vi "Test Lookup API.vi"() -> (0 "test result":errorcluster)   [LabVIEW 2019, in "ANODE Tests.lvlib"]
uses:
  ANODE Tests.lvlib
  Base Class A.lvclass
  Class B-D.lvclass
  C:/Users/Nicholas Folse/Documents/workspace/github-tauterra.llc/ANODE/ANODE Tests/Lookup API/Class B.lvclass
  Class B.lvclass
  C:/Users/Nicholas Folse/Documents/workspace/github-tauterra.llc/ANODE/ANODE Tests/Lookup API/Base Class A.lvclass
  208e85c7-0cb6-4da8-adaf-c1f07bea2b81.vi
  350f7c64-ba5b-4f87-a26e-5058ffd36ae8.vi
  9f842d0e-53a4-4d11-badb-58d219860510.vi
  80fdccb2-9c7f-43c5-aac1-790debc25787.vi
  208e85c7-0cb6-4da8-adaf-c1f07bea2b81.vi/252e9e58-4af6-4f6d-a0ca-3bfdda4348ce.vi
  350f7c64-ba5b-4f87-a26e-5058ffd36ae8.vi/97c9d0db-94a5-468f-a424-c7048e2c2629.vi
  9f842d0e-53a4-4d11-badb-58d219860510.vi/c3dc75b2-7c32-4953-a8c5-a3642948c66d.vi
  ANODE/Lookup API/Services/Lookup Service/Lookup Service.lvclass
  Class C.lvclass
  1f8dec34-990c-434d-8cda-825a1ce43037.vi
panel:
  out "should have two instances of 'A'":bool
  out "error out":errorcluster
  out "pass?":bool
  out "object should be in set":bool
  out "B and B-C instance are both 'A's":bool
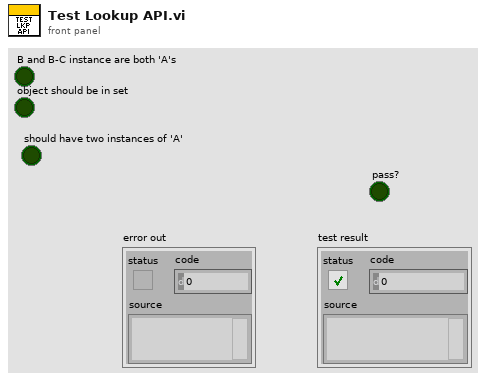
[diagram p1: front panel]
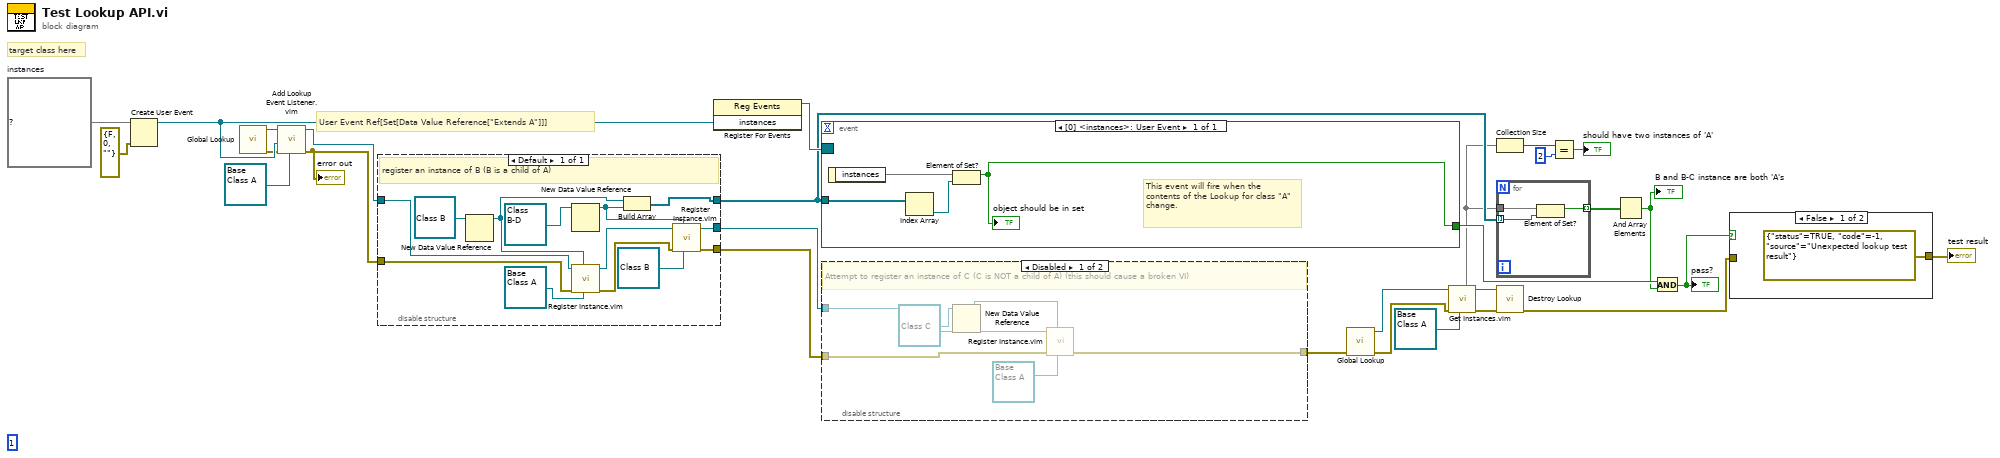
[diagram p0: block diagram]
diagram:
  (unwired) 1
  w13 = set{refnum<data-value>} {}  # instances
  # "User Event Ref[Set[Data Value Reference[\"Extends A\"]]]"
  # "target class here"
  n1 = Create User Event(user event datatype=w13, error in=errorcluster {"status"=FALSE, "code"=0, "source"=""} ("error in (no error)")) -> (user event=w12:refnum<user-event>)  [unwired: 1 out]
  n2 = call "Global Lookup.vi"() -> ("error out"=w8:errorcluster, "Global Lookup"=w15:refnum<data-value>)  [unwired: 10 in]
  n3 = call "Add Lookup Event Listener.vim"("Base Class (LabVIEW Object)"=refnum<class "Base Class A.lvclass"> refnum ("LVCOOOP Tests.lvlib:Base Class A.lvclass"), "error in (no error)"=w8, "user event"=w12, "Lookup Service in"=w15) -> ("error out"=w10:errorcluster, "Lookup Service out"=w11:refnum<data-value>)  [unwired: 6 in]
  "error out" <- w10
  n4 = disable-structure shown="Default" {
    disable-tunnel: w11 -> [w40]
    disable-tunnel: [w33] -> w27
    disable-tunnel: w10 -> [w39]
    disable-tunnel: [w32] -> w19
    disable-tunnel: [w29] -> w6
    frame Enabled {
      # "register an instance of B (B is a child of A)"
      n5 = New Data Value Reference(data value=refnum<class "Class B.lvclass"> refnum ("LVCOOOP Tests.lvlib:Class B.lvclass")) -> (data value reference=w31:refnum<data-value>)  [unwired: 1 in, 1 out]
      n6 = New Data Value Reference(data value=refnum<class "Class B-D.lvclass"> refnum ("LVCOOOP Tests.lvlib:Class B-D.lvclass")) -> (data value reference=w30:refnum<data-value>)  [unwired: 1 in, 1 out]
      n7 = call "Register Instance.vim"("Base Class (LabVIEW Object)"=refnum<class "Base Class A.lvclass"> refnum ("LVCOOOP Tests.lvlib:Base Class A.lvclass"), "Object Instance"=w31, "error in (no error)"=w39, "Lookup Service in"=w40) -> ("error out"=w36:errorcluster, "Lookup Service out"=w37:refnum<data-value>)  [unwired: 6 in]
      n8 = Build Array(w31, w30) -> (w29:refnum<data-value>[])
      n9 = call "Register Instance.vim"("Base Class (LabVIEW Object)"=refnum<class "Class B.lvclass"> refnum ("LVCOOOP Tests.lvlib:Class B.lvclass"), "Object Instance"=w30, "error in (no error)"=w36, "Lookup Service in"=w37) -> ("error out"=w32:errorcluster, "Lookup Service out"=w33:refnum<data-value>)  [unwired: 6 in]
    }
  }
  n10 = register-events(w12) -> (reference out=w28:refnum<event-registration>)  [unwired: 2 in, 1 out]
  n11 = event shown="[0] <instances>: User Event" {
    selector: w28 -> [_]
    dyn-events: _ -> [_]
    timeout: _ -> [_]
    tunnel: [w42] -> w24
    tunnel: w6 -> [w44]
    event User Event {
      # "This event will fire when the contents of the Lookup for class \"A\" change."
      n12 = event-data() -> ("instances"=w45:set{refnum<data-value>})  [unwired: 1 in]
      n13 = Index Array(array=w44) -> (element=w43:refnum<data-value>)  [unwired: 1 in]
      n14 = Element of Set?(10:w43, 11:w45) -> (3:w42:bool)
      "object should be in set" <- w42
    }
  }
  n15 = disable-structure shown="Disabled" {
    disable-tunnel: w27 -> [w51 _]
    disable-tunnel: w19 -> [w49 w52]
    disable-tunnel: [w46 w52] -> w18
    frame Disabled {
      # "Attempt to register an instance of C (C is NOT a child of A) (this should cause a broken VI)"
      n16 = New Data Value Reference(data value=refnum<class "Class C.lvclass"> refnum ("LVCOOOP Tests.lvlib:Class C.lvclass")) -> (data value reference=w47:refnum<data-value>)  [unwired: 1 in, 1 out]
      n17 = call "Register Instance.vim"("Base Class (LabVIEW Object)"=refnum<class "Base Class A.lvclass"> refnum ("LVCOOOP Tests.lvlib:Base Class A.lvclass"), "Object Instance"=w47, "error in (no error)"=w49, "Lookup Service in"=w51) -> ("error out"=w46:errorcluster)  [unwired: 6 in, 1 out]
    }
    frame Enabled {
    }
  }
  n18 = call "Global Lookup.vi"("error in (no error)"=w18) -> ("error out"=w17:errorcluster, "Global Lookup"=w16:refnum<data-value>)  [unwired: 9 in]
  n19 = call "Get Instances.vim"("Base Class (LabVIEW Object)"=refnum<class "Base Class A.lvclass"> refnum ("LVCOOOP Tests.lvlib:Base Class A.lvclass"), "error in (no error)"=w17, "Lookup Service in"=w16) -> ("error out"=w25:errorcluster, "Lookup Service out"=w26:refnum<data-value>, "instances"=w4:set{refnum<data-value>})  [unwired: 6 in]
  n20 = Collection Size(1:w4) -> (0:w3:i32)
  n21 = for {
    tunnel: w4 -> [w55]
    tunnel: w6 -> [w54] mode=indexing
    tunnel: [w53] -> w7 mode=indexing
    n22 = Element of Set?(10:w54, 11:w55) -> (3:w53:bool)
  }
  n23 = call "Destroy Lookup.vi"("error in (no error)"=w25, "Lookup Service in"=w26) -> ("error out"=w21:errorcluster)  [unwired: 8 in, 1 out]
  n24 = Equal?(x=w3, y=2) -> (x = y?=→"should have two instances of 'A'":bool)
  n25 = And Array Elements(Boolean array=w7) -> (logical AND=w5:bool)
  "B and B-C instance are both 'A's" <- w5
  n26 = And(x=w24, y=w5) -> (x .and. y?=w23:bool)
  "pass?" <- w23
  n27 = case shown="False" w23 {
    tunnel: [errorcluster {"status"=TRUE, "code"=-1, "source"="Unexpected lookup test result"} ("test result") w57] -> w22
    tunnel: w21 -> [_ w57]
    frame False {
    }
    frame True {
    }
  }
  "test result" <- w22
